vi "Convert Bitfile Data to RingTypeDef Data.vi"(8 "error in":errorcluster, 10 "FIFOs":cluster{"HostToTargetFIFOs":T1[]}[](array[cluster]), 11 "Registers":cluster{"Controls":T3[]}[](array[cluster])) -> (0 "error out":errorcluster, 3 "TypeDef Info":cluster{string, string[]}[](array[cluster]))   [LabVIEW 2010]
uses:
  <userlib>/_FPGA Interface Advanced Tools/FPGA Bitfile Utility/TypeDefs/Control_Indicator Info.ctl
  <vilib>/rvi/DataTransferAndStorage/Container/Common/niFpgaDataTypeControl.ctl
  <userlib>/_FPGA Interface Advanced Tools/FPGA Bitfile Utility/TypeDefs/FIFO Info.ctl
  <userlib>/_FPGA Interface Advanced Tools/FPGA Bitfile Utility/FPGA Bitfile Utility.lvlib
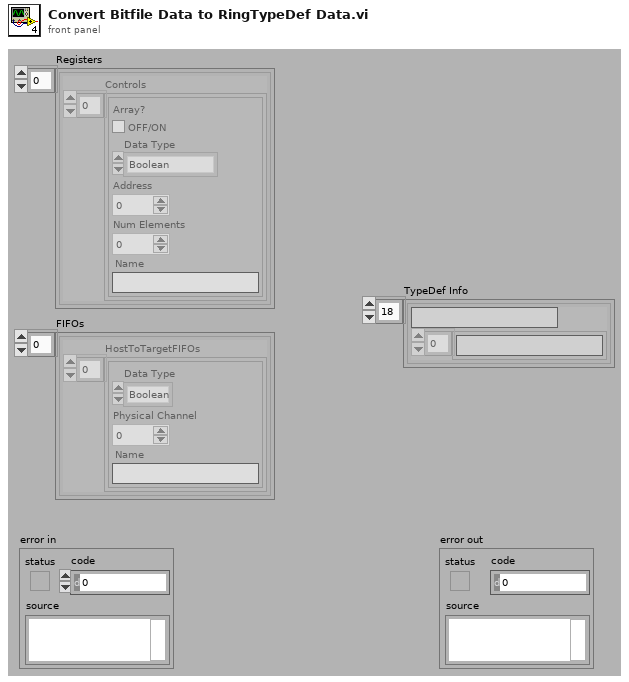
[diagram p1: front panel]
types:
  T1 = typedef "FPGA Bitfile Utility.lvlib/FIFO Info.ctl" = cluster{"Data Type":T2, "Physical Channel":u32, "Name":string}
  T2 = typedef "niFpgaDataTypeControl.ctl" = enum32{"Boolean", "I8", "I16", "I32", "I64", "U8", "U16", "U32", "U64", "FXP", "CustomControl"}
  T3 = typedef "FPGA Bitfile Utility.lvlib/Control_Indicator Info.ctl" = cluster{"Array?":bool, "Data Type":T2, "Address":u32, "Num Elements":u32, "Name":string}
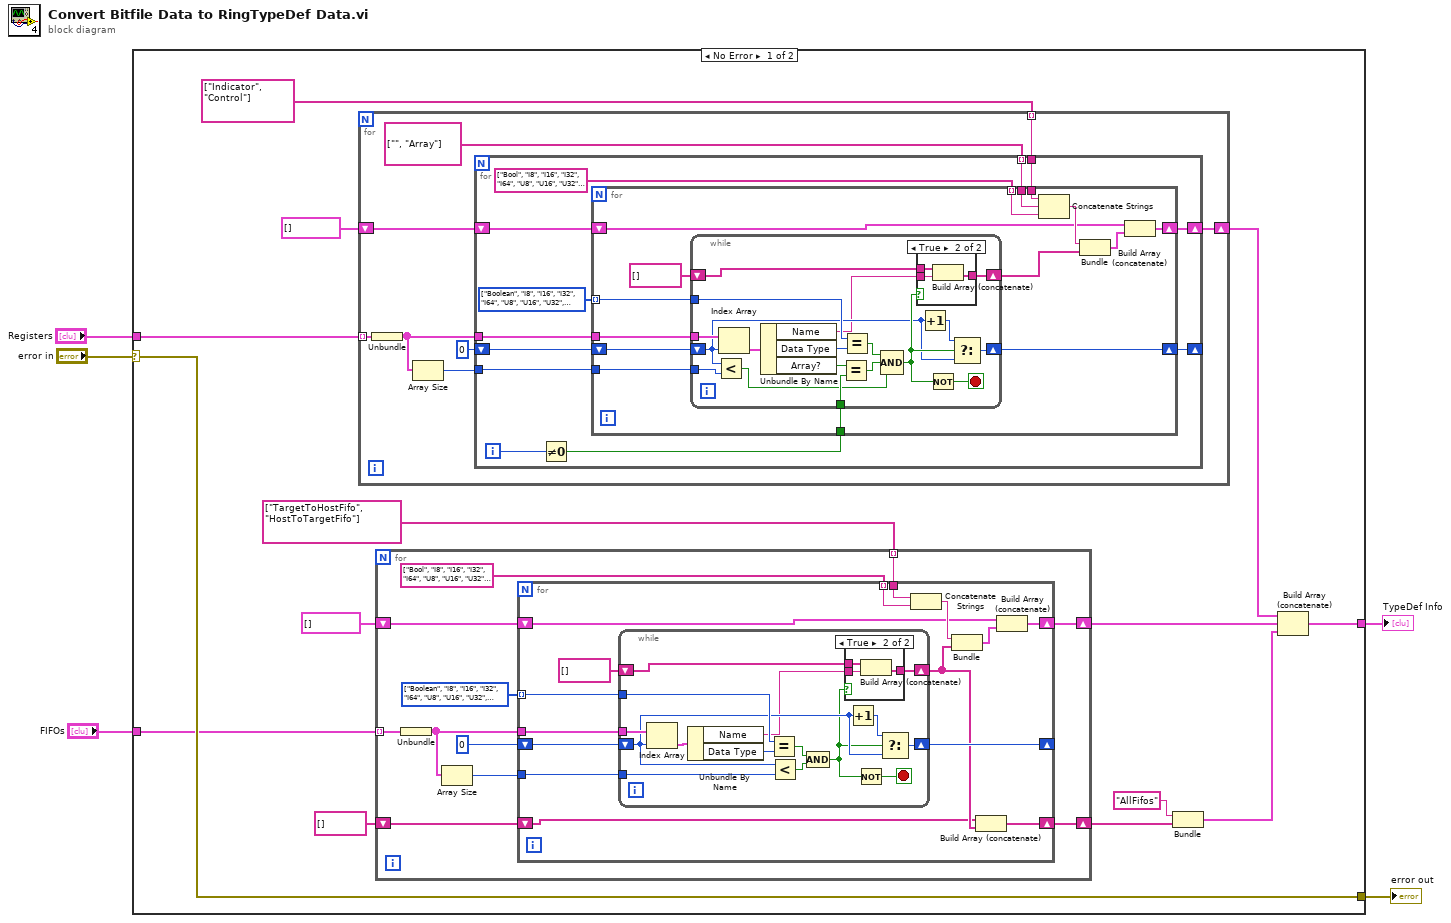
[diagram p0: block diagram]
diagram:
  n1 = case shown="No Error" "error in" {
    selector: "error in" -> [w13 w122]
    tunnel: [w14 _] -> w5
    tunnel: [w13 w122] -> w4
    tunnel: "Registers" -> [w11 _]
    tunnel: "FIFOs" -> [w10 _]
    frame No Error {
      n2 = for {
        tunnel: w11 -> [w72] mode=indexing
        tunnel: string[] ["Indicator", "Control"] -> [w70] mode=indexing
        shift-right: [w69] -> w16
        shift-left: cluster{string, string[]}[] [] -> [w68]
        n3 = Unbundle(w72) -> ("Controls"=w66:T3[])
        n4 = Array Size(array=w66) -> (size(s)=w65:i32)
        n5 = for {
          tunnel: w66 -> [w84]
          shift-right: [w81] -> _
          shift-left: 0 -> [w82]
          tunnel: string[] ["", "Array"] -> [w76] mode=indexing
          tunnel: w70 -> [w77]
          shift-right: [w75] -> w69
          shift-left: w68 -> [w74]
          tunnel: w65 -> [w73]
          i -> [w83]
          w79 = T2[] [enum."Boolean", enum."I8", enum."I16", enum."I32", enum."I64", enum."U8", enum."U16", enum."U32", enum."U64"] items=["Boolean", "I8", "I16", "I32", "I64", "U8", "U16", "U32", "U64", "FXP", "CustomControl"]
          n6 = Not Equal To 0?(x=w83) -> (x != 0?=w80:bool)
          n7 = for {
            tunnel: w79 -> [w99] mode=indexing
            tunnel: w84 -> [w98]
            tunnel: w80 -> [w95]
            shift-right: [w96] -> w81
            shift-left: w82 -> [w97]
            tunnel: string[] ["Bool", "I8", "I16", "I32", "I64", "U8", "U16", "U32", "U64"] -> [w90] mode=indexing
            tunnel: w77 -> [w92]
            tunnel: w76 -> [w91]
            shift-right: [w87] -> w75
            shift-left: w74 -> [w86]
            tunnel: w73 -> [w85]
            n8 = while {
              tunnel: w99 -> [w111]
              tunnel: w98 -> [w117]
              shift-right: [w115] -> w96
              shift-left: w97 -> [w103]
              tunnel: w95 -> [w113]
              shift-right: [w104] -> w93
              shift-left: string[] [] -> [w105]
              tunnel: w85 -> [w102]
              stop <- w106 stop-if-true
              n9 = Less?(x=w103, y=w102) -> (x < y?=w101:bool)
              n10 = Index Array(array=w117, index=w103) -> (element=w108:T3)
              n11 = Unbundle By Name(w108) -> ("Name"=w100:string, "Data Type"=w112:T2, "Array?"=w114:bool)
              n12 = Equal?(x=w114, y=w113) -> (x = y?=w110:bool)
              n13 = Equal?(x=w111, y=w112) -> (x = y?=w109:bool)
              n14 = Compound Arithmetic op=AND(w109, w110, w101) -> (w107:bool)
              n15 = case shown="True" w107 {
                tunnel: w105 -> [w118 w121]
                tunnel: w100 -> [_ w120]
                tunnel: [w118 w119] -> w104
                frame False {
                }
                frame True {
                  n16 = Build Array (concatenate)(w121, w120) -> (w119:string[])
                }
              }
              n17 = Increment(x=w103) -> (x+1=w116:i32)
              n18 = Not(x=w107) -> (.not. x?=w106:bool)
              n19 = Select(t=w116, s=w107, f=w103) -> (s? t:f=w115:i32)
            }
            n20 = Concatenate Strings(w92, w91, w90) -> (w89:string)
            n21 = Bundle(w89, w93) -> (w88:cluster{string, string[]})  [unwired: 1 in]
            n22 = Build Array (concatenate)(w86, w88) -> (w87:cluster{string, string[]}[])
          }
        }
      }
      n23 = for {
        tunnel: w10 -> [w30] mode=indexing
        shift-right: [w29] -> w15
        shift-left: cluster{string, string[]}[] [] -> [w28]
        tunnel: string[] ["TargetToHostFifo", "HostToTargetFifo"] -> [w25] mode=indexing
        shift-right: [w21] -> w8
        shift-left: string[] [] -> [w20]
        w27 = T2[] [enum."Boolean", enum."I8", enum."I16", enum."I32", enum."I64", enum."U8", enum."U16", enum."U32", enum."U64"] items=["Boolean", "I8", "I16", "I32", "I64", "U8", "U16", "U32", "U64", "FXP", "CustomControl"]
        n24 = Unbundle(w30) -> ("HostToTargetFIFOs"=w22:T1[])
        n25 = Array Size(array=w22) -> (size(s)=w23:i32)
        n26 = for {
          tunnel: w27 -> [w45] mode=indexing
          tunnel: w22 -> [w44]
          shift-right: [w42] -> _
          shift-left: 0 -> [w43]
          tunnel: string[] ["Bool", "I8", "I16", "I32", "I64", "U8", "U16", "U32", "U64"] -> [w39] mode=indexing
          tunnel: w25 -> [w40]
          shift-right: [w36] -> w29
          shift-left: w28 -> [w35]
          tunnel: w23 -> [w34]
          shift-right: [w32] -> w21
          shift-left: w20 -> [w31]
          n27 = while {
            tunnel: w45 -> [w56]
            tunnel: w44 -> [w60]
            shift-right: [w58] -> w42
            shift-left: w43 -> [w50]
            shift-right: [w52] -> w33
            shift-left: string[] [] -> [w53]
            tunnel: w34 -> [w51]
            stop <- w54 stop-if-true
            n28 = Index Array(array=w60, index=w50) -> (element=w55:T1)
            n29 = Unbundle By Name(w55) -> ("Name"=w46:string, "Data Type"=w57:T2)
            n30 = Equal?(x=w56, y=w57) -> (x = y?=w48:bool)
            n31 = Less?(x=w50, y=w51) -> (x < y?=w49:bool)
            n32 = Compound Arithmetic op=AND(w48, w49) -> (w47:bool)
            n33 = case shown="True" w47 {
              tunnel: w53 -> [w61 w64]
              tunnel: w46 -> [_ w63]
              tunnel: [w61 w62] -> w52
              frame False {
              }
              frame True {
                n34 = Build Array (concatenate)(w64, w63) -> (w62:string[])
              }
            }
            n35 = Increment(x=w50) -> (x+1=w59:i32)
            n36 = Not(x=w47) -> (.not. x?=w54:bool)
            n37 = Select(t=w59, s=w47, f=w50) -> (s? t:f=w58:i32)
          }
          n38 = Concatenate Strings(w40, w39) -> (w38:string)
          n39 = Bundle(w38, w33) -> (w37:cluster{string, string[]})  [unwired: 1 in]
          n40 = Build Array (concatenate)(w31, w33) -> (w32:string[])
          n41 = Build Array (concatenate)(w35, w37) -> (w36:cluster{string, string[]}[])
        }
      }
      n42 = Bundle("AllFifos", w8) -> (w6:cluster{string, string[]})  [unwired: 1 in]
      n43 = Build Array (concatenate)(w16, w15, w6) -> (w14:cluster{string, string[]}[])
    }
    frame Error {
    }
  }
  "TypeDef Info" <- w5
  "error out" <- w4
